vi "setEdgeTrigger.vi"(7 "Source":string, 8 "error in (no error)":errorcluster, 9 "Edge":T1, 10 "Threshold [V]":dbl, 11 "ScopeNi in":refnum<class "ScopeNi.lvclass">) -> (0 "error out":errorcluster, 3 "ScopeNi out":refnum<class "ScopeNi.lvclass">)   [LabVIEW 2023, in "ScopeNi.lvclass"]
doc: "<b>Author:</b> Wolfgang\n<b>Description:</b> Configure Edge Trigger."
uses:
  ScopeNi.lvclass
  Data/scopeEdgeTrigger.ctl
  ScopeNi.lvclass/ScopeNi.ctl
  <instrlib>/niScope/Controls/niScope trigger slope.ctl
  <instrlib>/niScope/Configure/Trigger/niScope Configure Trigger Edge.vi
  sweScope.lvlib
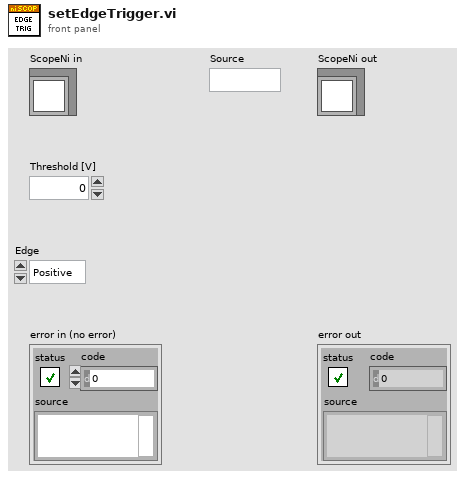
[diagram p1: front panel]
types:
  T1 = typedef "sweScope.lvlib/scopeEdgeTrigger.ctl" = enum16{"Positive", "Negative", "Either"}
  T2 = typedef "niScope trigger slope.ctl" = i32
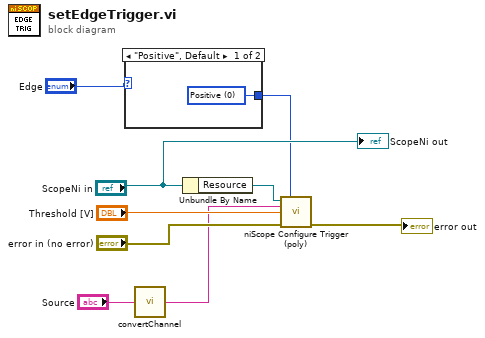
[diagram p0: block diagram]
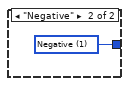
[diagram p2: hidden frame]
diagram:
  n1 = case shown="\"Positive\", Default" "Edge" {
    tunnel: [w10 w11] -> w3
    frame "Positive", Default {
      w10 = T2 0 items=["Positive", "Negative"] ("trigger slope")
    }
    frame "Negative" {
      w11 = T2 1 items=["Positive", "Negative"] ("trigger slope")
    }
  }
  n2 = call "convertChannel.vi"("Chn in"="Source") -> ("Chn out"=w1:string)
  n3 = Unbundle By Name("ScopeNi in") -> ("Resource"=w6:refnum<k15>)
  n4 = call-poly <instrlib>:"niScope Configure Trigger (poly).vi"("instrument handle"=w6, "trigger slope"=w3, "trigger source"=w1, "trigger level"="Threshold [V]", "error in"="error in (no error)") -> ("error out"=→"error out":errorcluster)  [unwired: 9 in, 1 out]
  "ScopeNi out" <- "ScopeNi in"
